vi "Upload to Cloud.vi"(8 "error in (no error)":errorcluster, 10 "Extra Comments":string, 11 "Zip File Path":path) -> (0 "error out":errorcluster)   [LabVIEW 2014, in "Raspberry Pi Compatible Compiler for LabVIEW.lvlib"]
uses:
  <vilib>/National Instruments/LabVIEW Interface for Amazon S3/Typedefs/AMZ_S3_AWS Credentials.ctl
  <vilib>/National Instruments/LabVIEW Interface for Amazon S3/Typedefs/AMZ_S3_Object Metadata.ctl
  <vilib>/National Instruments/LabVIEW Interface for Amazon S3/Typedefs/AMZ_S3_API_PUT Object Request Parameters.ctl
  <vilib>/National Instruments/LabVIEW Interface for Amazon S3/Typedefs/AMZ_S3_ACL.ctl
  <vilib>/National Instruments/LabVIEW Interface for Amazon S3/Typedefs/AMZ_S3_Storage Class.ctl
  <vilib>/National Instruments/LabVIEW Interface for Amazon S3/Typedefs/AMZ_S3_API_POST Multipart Object Request Parameters.ctl
  Raspberry Pi Compatible Compiler for LabVIEW.lvlib
  <vilib>/National Instruments/LabVIEW Interface for Amazon S3/LV Interface for Amazon S3.lvlib
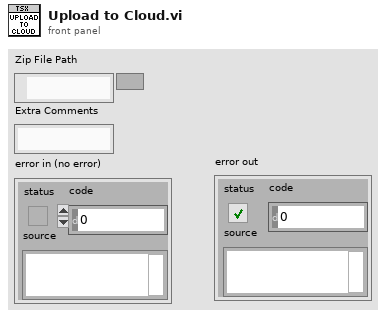
[diagram p1: front panel]
types:
  T1 = typedef "LV Interface for Amazon S3.lvlib/AMZ_S3_AWS Credentials.ctl" = cluster{"Access Key":string, "Secret Key":string}
  T2 = typedef "LV Interface for Amazon S3.lvlib/AMZ_S3_Object Metadata.ctl" = cluster{"Key":string, "Value":string}
  T3 = typedef "LV Interface for Amazon S3.lvlib/AMZ_S3_ACL.ctl" = enum16{"private", "public-read", "public-read-write", "authenticated-read", "bucket-owner-read", "bucket-owner-full-control"}
  T4 = typedef "LV Interface for Amazon S3.lvlib/AMZ_S3_API_PUT Object Request Parameters.ctl" = cluster{"Content Type":string, "ACL":T3, "Storage Class":T5, "User Metadata":T2[], "Content MD5":string}
  T5 = typedef "LV Interface for Amazon S3.lvlib/AMZ_S3_Storage Class.ctl" = enum16{"STANDARD", "REDUCED_REDUNDANCY"}
  T6 = typedef "LV Interface for Amazon S3.lvlib/AMZ_S3_API_POST Multipart Object Request Parameters.ctl" = cluster{"Content Type":string, "ACL":T3, "Storage Class":T5, "User Metadata":T2[]}
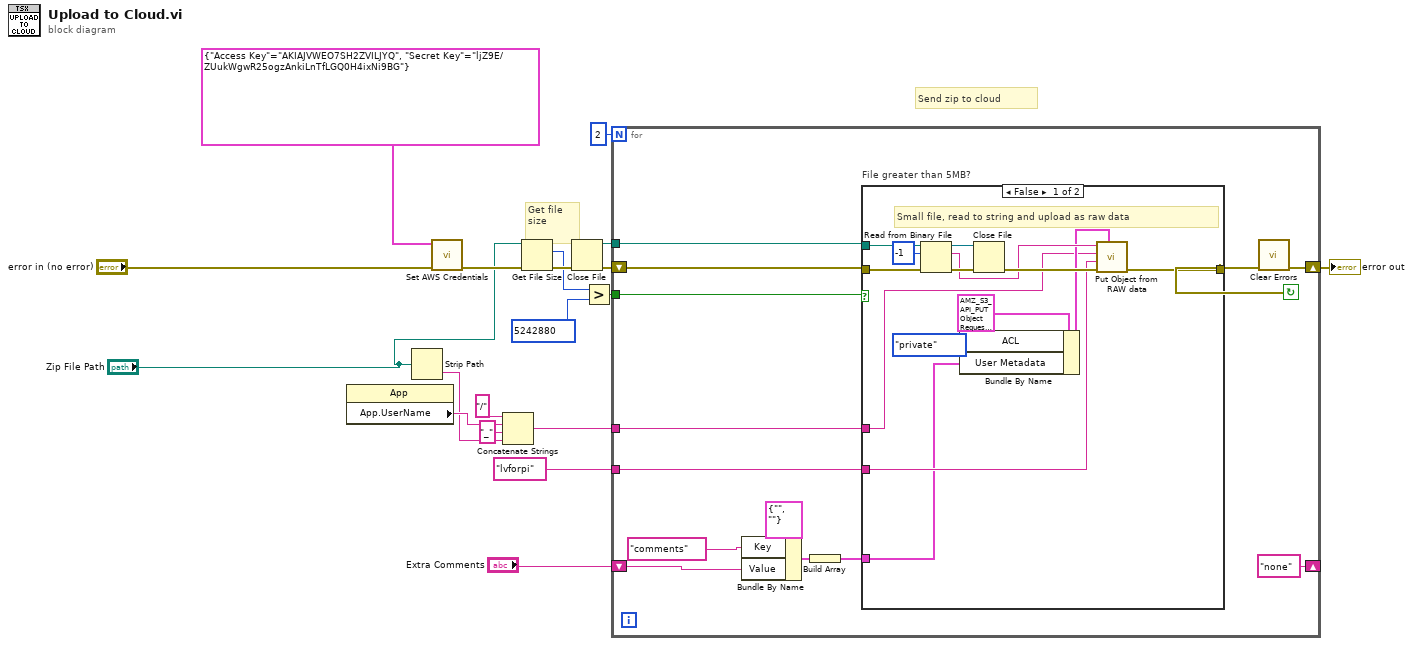
[diagram p0: block diagram]
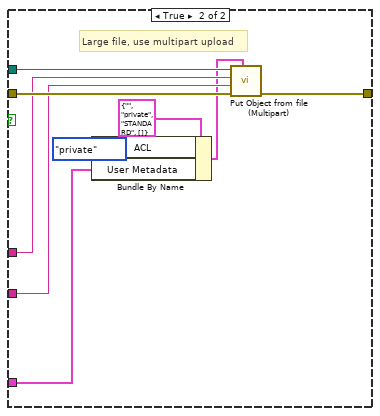
[diagram p2: hidden frame]
diagram:
  # "Get file\nsize"
  # "Send zip to cloud"
  n1 = property class="App"() -> ("App.UserName"=w10:string)  [unwired: 2 in, 2 out]
  n2 = Strip Path(path="Zip File Path") -> (name=w8:string)  [unwired: 1 out]
  n3 = call <vilib>:"Set AWS Credentials.vi"("error in (no error)"="error in (no error)", "AWS Credentials in"=T1 {"Access Key"="AKIAJVWEO7SH2ZVILJYQ", "Secret Key"="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"}) -> ("error out"=w12:errorcluster)  [unwired: 9 in]
  n4 = Concatenate Strings("/" ("string"), w10, "_" ("string"), w8) -> (w9:string)
  n5 = Get File Size(file="Zip File Path", error in=w12) -> (refnum out=w18:refnum<file>, size (in bytes)=w17:i64, 0:w19:errorcluster)
  n6 = Close File(refnum=w18, error in=w19) -> (path=w13:path, error out=w14:errorcluster)
  n7 = Greater?(x=w17, y=i64 5242880) -> (0:w15:bool)
  n8 = for {
    N: 2 -> [_]
    tunnel: w15 -> [w33]
    tunnel: w13 -> [w31]
    tunnel: w9 -> [w30]
    tunnel: "lvforpi" -> [w29]
    shift-right: [w28] -> w2
    shift-left: w14 -> [w32]
    shift-right: ["none" ("result string")] -> _
    shift-left: "Extra Comments" -> [w22]
    stop <- w26 continue-if-true
    n9 = Bundle By Name(cluster=T2 {"Key"="", "Value"=""} ("Object Metadata"), "Key"="comments", "Value"=w22) -> (w23:T2)
    n10 = Build Array(w23) -> (w21:T2[])
    n11 = case "File greater than 5MB?" shown="False" w33 {
      tunnel: w32 -> [w47 w56]
      tunnel: w31 -> [w46 w55]
      tunnel: w29 -> [w37 w53]
      tunnel: w30 -> [w36 w54]
      tunnel: [w38 w52] -> w26
      tunnel: w21 -> [w34 w48]
      frame False {
        # "Small file, read to string and upload as raw data"
        n12 = Read from Binary File(8:w47, 10:-1 ("count (1)"), 11:w46) -> (0:w44:errorcluster, 2:w41:string, 3:w43:refnum<file>)  [unwired: 3 in, 1 out]
        n13 = Bundle By Name(cluster=T4 {"Content Type"="", "ACL"=enum."private", "Storage Class"=enum."STANDARD", "User Metadata"=[], "Content MD5"=""} ("Request Parameters"), "ACL"=AMZ_S3_ACL."private", "User Metadata"=w34) -> (w39:T4)
        n14 = Close File(refnum=w43, error in=w44) -> (error out=w42:errorcluster)  [unwired: 1 out]
        n15 = call <vilib>:"Put Object from RAW data.vi"("Request Parameters"=w39, "error in (no error)"=w42, "Bucket"=w37, "Path"=w36, "Data"=w41) -> ("error out"=w38:errorcluster)  [unwired: 5 in, 1 out]
      }
      frame True {
        # "Large file, use multipart upload"
        n16 = Bundle By Name(cluster=T6 {"Content Type"="", "ACL"=enum."private", "Storage Class"=enum."STANDARD", "User Metadata"=[]} ("Request Parameters"), "ACL"=AMZ_S3_ACL."private", "User Metadata"=w48) -> (w50:T6)
        n17 = call <vilib>:"Put Object from file (Multipart).vi"("Request Parameters"=w50, "error in (no error)"=w56, "Bucket"=w53, "Object path"=w54, "Local file path"=w55) -> ("error out"=w52:errorcluster)  [unwired: 4 in, 2 out]
      }
    }
    n18 = call <vilib>:"Clear Errors.vi"("error in (no error)"=w26) -> ("error out"=w28:errorcluster)  [unwired: 5 in, 1 out]
  }
  "error out" <- w2
